vi "Get Acquisition Type.vi"(8 "error in (no error)":errorcluster, 11 "VISA resource name":refnum<visa-resource-name>) -> (0 "error out":errorcluster, 2 "Acquisition Type":i32, 3 "VISA resource name out":refnum<visa-resource-name>)   [LabVIEW 2011, in "Agilent DSO1000 Series.lvlib"]
doc: "This VI reads how the oscilloscope accquires data and fills the waveform record."
uses:
  <instrlib>/Agilent DSO1000 Series/Agilent DSO1000 Series.lvlib
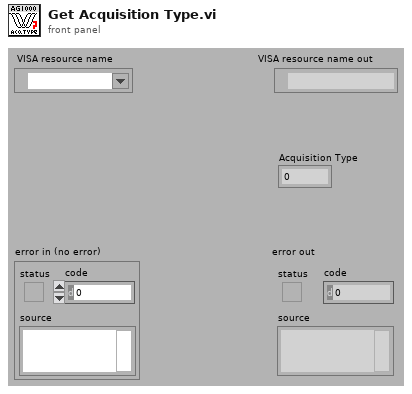
[diagram p1: front panel]
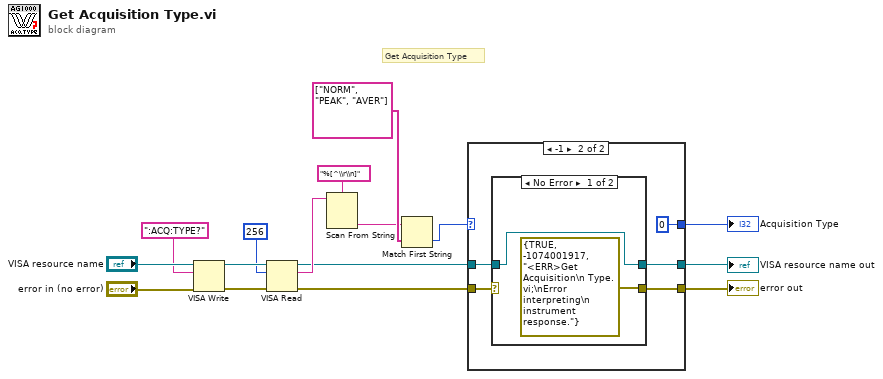
[diagram p0: block diagram]
diagram:
  # "Get Acquisition Type"
  n1 = VISA Write(VISA resource name="VISA resource name", write buffer=":ACQ:TYPE?", error in (no error)="error in (no error)") -> (VISA resource name out=w13:refnum<visa-resource-name>, error out=w12:errorcluster)  [unwired: 1 out]
  n2 = VISA Read(VISA resource name=w13, byte count=u32 256, error in (no error)=w12) -> (VISA resource name out=w8:refnum<visa-resource-name>, read buffer=w10:string, error out=w7:errorcluster)  [unwired: 1 out]
  n3 = Scan From String(format string="%[^\\r\\n]", input string=w10) -> (output 1=w2:string)  [unwired: 3 in, 3 out]
  n4 = Match First String(2:string[] ["NORM", "PEAK", "AVER"] ("1D array"), 3:w2) -> (0:w1:i32)  [unwired: 1 out]
  n5 = case shown="-1" w1 {
    selector: w1 -> [w19 _]
    tunnel: w8 -> [w18 w23]
    tunnel: w7 -> [w17 w24]
    tunnel: [w18 w22] -> w6
    tunnel: [w17 w21] -> w5
    tunnel: [w19 0 ("index of element")] -> w4
    frame 0, Default {
    }
    frame -1 {
      n6 = case shown="No Error" w24 {
        selector: w24 -> [_ w28]
        tunnel: w23 -> [w25 w27]
        tunnel: [errorcluster {TRUE, -1074001917, "<ERR>Get Acquisition\n Type.vi;\nError interpreting\n instrument response."} w28] -> w21
        tunnel: [w25 w27] -> w22
        frame No Error {
        }
        frame Error {
        }
      }
    }
  }
  "VISA resource name out" <- w6
  "error out" <- w5
  "Acquisition Type" <- w4
